vi "SN_TcpConnectRef.vi"() -> ()   [LabVIEW 2015]
panel:
  in  "Connect":refnum<vi>[](array[refnum])
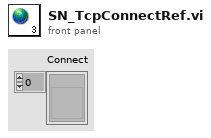
[diagram p1: front panel]
diagram:
